vi "定点周期设置.vi"(7 "Display State In":T1={"仪器状态"=FALSE, "仪器时间"=timestamp(0 s since 1904-01-01), "测量参数"={"氨氮"=TRUE, "总磷"=TRUE, "总氮"=TRUE, "CODMn"=TRUE, "CODCr"=FALSE}, "调用模块名称"="", "测试状态"={"启动时间"=timestamp(0 s since 1904-01-01), "结束时间"=timestamp(0 s since 1904-01-01), "启动次数"=0.0}}, 9 "间隔启动":T7, 10 "定点周期":T4, 11 "周期模式":T3) -> (2 "保存输出":bool, 3 "周期设置输出":T6={"周期模式"=enum."不启用", "测量参数"={"氨氮"=TRUE, "总磷"=TRUE, "总氮"=TRUE, "CODMn"=TRUE, "CODCr"=FALSE}, "定点周期"={"启动命令"=enum."", "启动命令 2"=enum."", "启动命令 3"=enum."", "启动命令 4"=enum."", "启动命令 5"=enum."", "启动命令 6"=enum."", "启动命令 7"=enum."", "启动命令 8"=enum."", "启动命令 9"=enum."", "启动命令 10"=enum."", "启动命令 11"=enum."", "启动命令 12"=enum."", "启动命令 13"=enum."", "启动命令 14"=enum."", "启动命令 15"=enum."", "启动命令 16"=enum."", "启动命令 17"=enum."", "启动命令 18"=enum."", "启动命令 19"=enum."", "启动命令 20"=enum."", "启动命令 21"=enum."", "启动命令 22"=enum."", "启动命令 23"=enum."", "启动命令 24"=enum.""}, "间隔设置"={"启动命令"=enum."", "启动间隔"=0.0, "启动次数"=0}})   [LabVIEW 2016, in "ZK定时设置.xctl"]
panel:
  out "测试状态.结束时间":timestamp caption="结束时间" format="%<%y/%m/%d %H:%M:%S>T"
  out "测试状态.启动次数":dbl caption="启动次数"
  out "测试状态.启动时间":timestamp caption="启动时间" format="%<%y/%m/%d %H:%M:%S>T"
  in  "测量参数":T2={"氨氮"=TRUE, "总磷"=TRUE, "总氮"=TRUE, "CODMn"=TRUE, "CODCr"=FALSE}
  in  "保存":bool
  in  "退出":bool
  in  "批量设置":bool
  out "周期模式选择卡":enum32{"选项卡 1", "选项卡 2"}(tab)
  # "分钟"
  # "次"
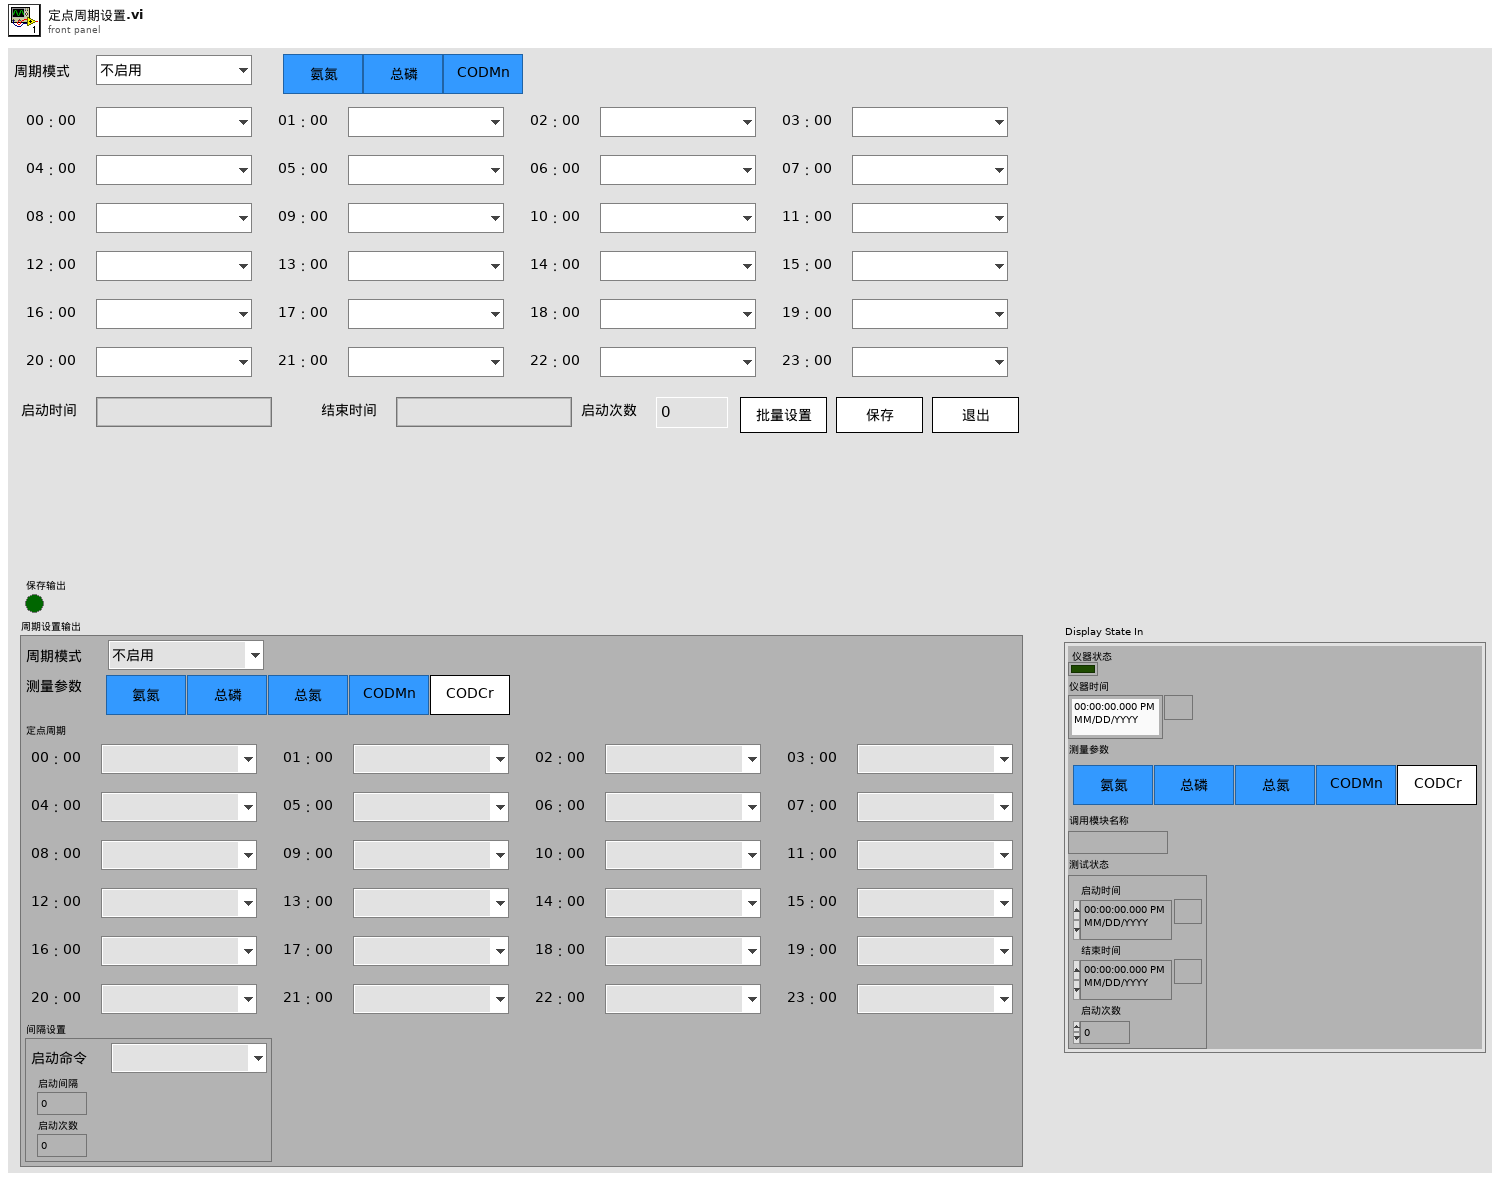
[diagram p1: front panel]
types:
  T1 = typedef "ZK定时设置.xctl/状态 1.ctl" = cluster{"仪器状态":bool, "仪器时间":timestamp, "测量参数":T2, "调用模块名称":string, "测试状态":cluster{"启动时间":timestamp, "结束时间":timestamp, "启动次数":dbl}}
  T2 = typedef "ZK定时设置.xctl/测量参数.ctl" = cluster{"氨氮":bool, "总磷":bool, "总氮":bool, "CODMn":bool, "CODCr":bool}
  T3 = typedef "ZK定时设置.xctl/周期模式设置.ctl" = enum16{"不启用", "定点模式", "间隔模式"}
  T4 = typedef "ZK定时设置.xctl/定点周期设置.ctl" = cluster{"启动命令":T5, "启动命令 2":T5, "启动命令 3":T5, "启动命令 4":T5, "启动命令 5":T5, "启动命令 6":T5, "启动命令 7":T5, "启动命令 8":T5, "启动命令 9":T5, "启动命令 10":T5, "启动命令 11":T5, "启动命令 12":T5, "启动命令 13":T5, "启动命令 14":T5, "启动命令 15":T5, "启动命令 16":T5, "启动命令 17":T5, "启动命令 18":T5, "启动命令 19":T5, "启动命令 20":T5, "启动命令 21":T5, "启动命令 22":T5, "启动命令 23":T5, "启动命令 24":T5}
  T5 = typedef "ZK定时设置.xctl/启动命令选择.ctl" = enum16{"", "加标回收（启动采配水）", "加标回收（不启动采配水）", "水样测试（启动采配水）", "水样测试（不启动采配水）", "平行样测试（启动采配水）", "平行样测试（不启动采配水）", "集成干预测试"}
  T6 = cluster{"周期模式":T3, "测量参数":T2, "定点周期":T4, "间隔设置":cluster{"启动命令":T5, "启动间隔":dbl, "启动次数":i32}}
  T7 = typedef "ZK定时设置.xctl/间隔启动设置.ctl" = cluster{"启动命令":T5, "启动间隔":dbl, "启动次数":i32}
  T8 = typedef "周期设置.lvlib/周期模式设置.ctl" = enum16{"不启用", "定点模式", "间隔模式"}
  T9 = cluster{"周期模式":T3, "测量参数":T2, "定点周期":T4, cluster{"启动命令":T5, "启动间隔":dbl, "启动次数":i32}}
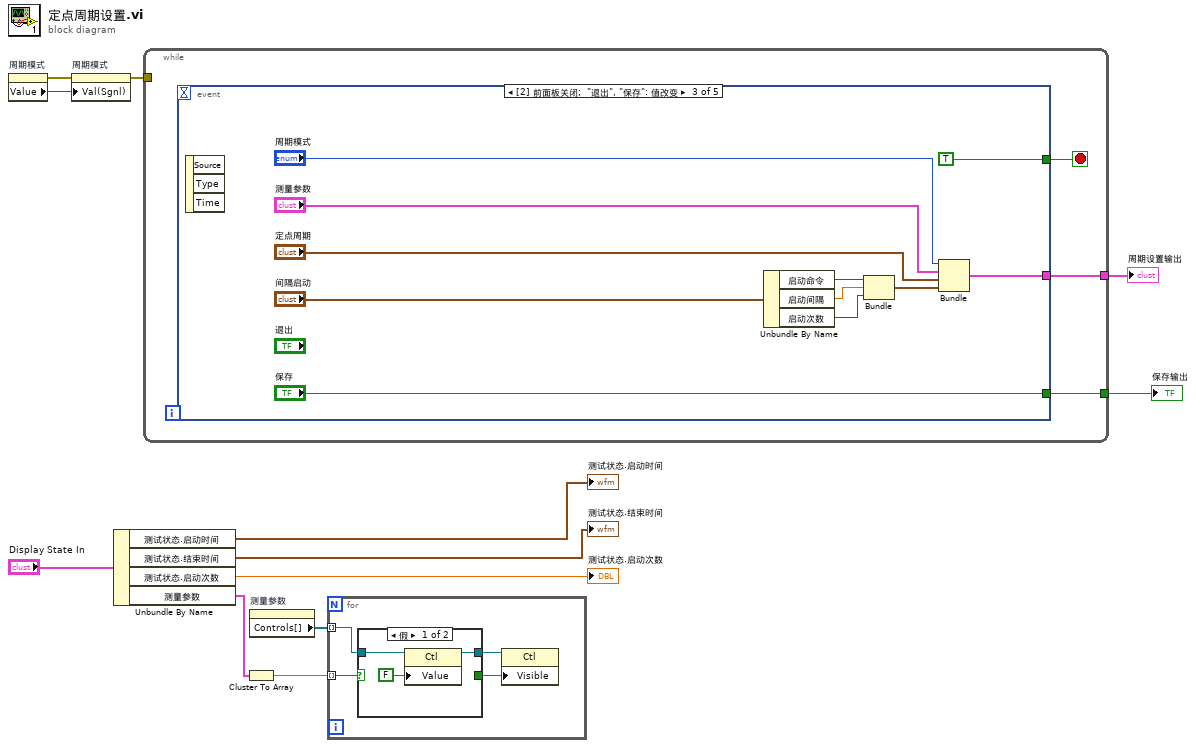
[diagram p0: block diagram]
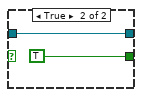
[diagram p2: hidden frame]
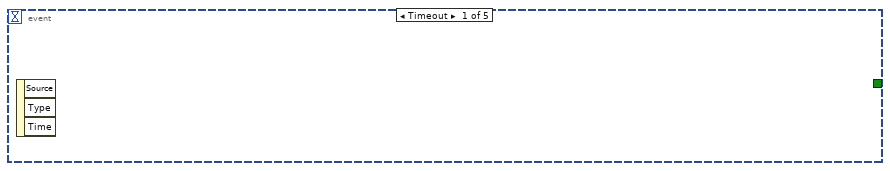
[diagram p3: hidden frame]
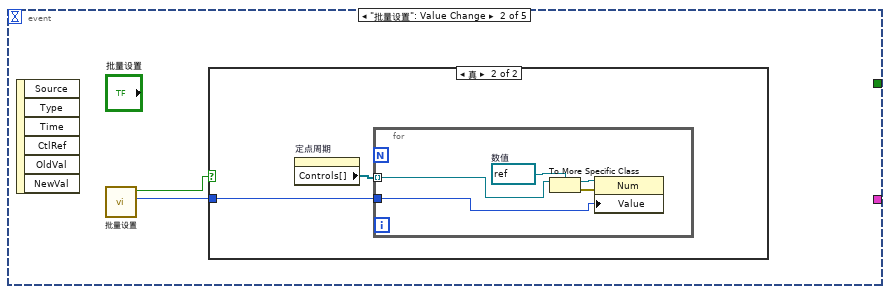
[diagram p4: hidden frame]
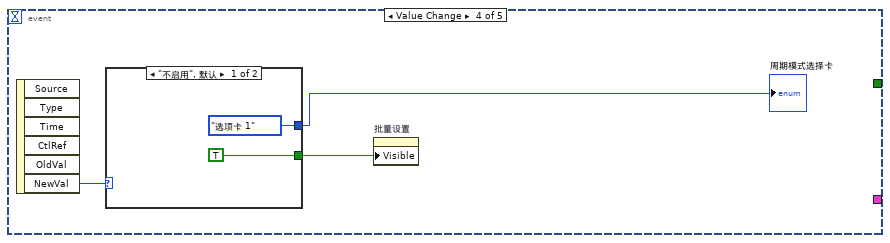
[diagram p6: hidden frame]
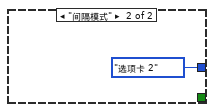
[diagram p7: hidden frame]
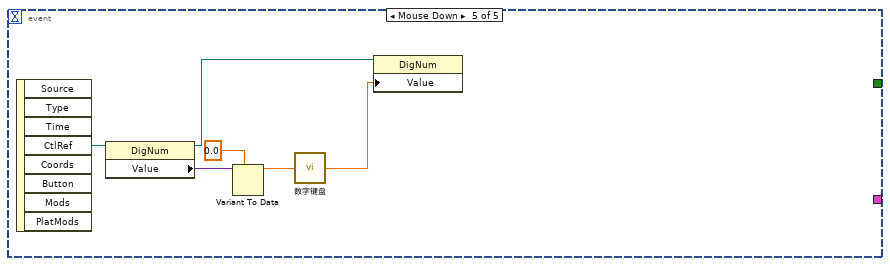
[diagram p8: hidden frame]
diagram:
  n1 = property on="周期模式" class="Enum (严格)"() -> (error out=w11:errorcluster, "Value"=w12:T8)  [unwired: 2 in, 1 out]
  n2 = property on="周期模式" class="Enum (严格)"(error in=w11, "Val(Sgnl)"=w12) -> (error out=w10:errorcluster)  [unwired: 1 in, 1 out]
  n3 = Unbundle By Name("Display State In") -> ("测试状态.启动时间"=→"测试状态.启动时间":timestamp, "测试状态.结束时间"=→"测试状态.结束时间":timestamp, "测试状态.启动次数"=→"测试状态.启动次数":dbl, "测量参数"=w1:T2)
  n4 = while {
    tunnel: [w14] -> w9
    tunnel: w10 -> [_]
    tunnel: [w13] -> w8
    stop <- w15 stop-if-true
    n5 = event shown="[2] 前面板关闭;  \"退出\", \"保存\": 值改变" {
      selector: _ -> [_ _ _ _ _]
      dyn-events: _ -> [_ _ _ _ _]
      timeout: _ -> [_ _ _ _ _]
      tunnel: [_ _ TRUE _ _] -> w15
      tunnel: [_ _ w34 _ _] -> w14
      tunnel: [_ _ "保存" _ _] -> w13
      event Timeout {
        n6 = event-data() -> ()  [unwired: 1 in, 3 out]
      }
      event "批量设置": Value Change {
        n7 = event-data() -> ()  [unwired: 1 in, 6 out]
        n8 = call "批量设置.vi"() -> ("启动命令 2"=w17:T5, "确定 2"=w16:bool)  [unwired: 10 in]
        n9 = case shown="真" w16 {
          tunnel: w17 -> [_ w18]
          frame False {
          }
          frame True {
            n10 = property on="定点周期" class="Clust (严格)"() -> ("Controls[]"=w19:refnum<vi>[])  [unwired: 2 in, 2 out]
            n11 = for {
              tunnel: w19 -> [w24] mode=indexing
              tunnel: w18 -> [w20]
              w23 = refnum<vi> refnum  # 数值
              n12 = To More Specific Class(target class=w23, reference=w24) -> (specific class reference=w22:refnum<vi>, error out=w21:errorcluster)  [unwired: 1 in]
              n13 = property class="Num"(reference=w22, error in=w21, "Value"=w20) -> ()  [unwired: 2 out]
            }
          }
        }
      }
      event Panel Close; "退出", "保存": Value Change {
        n14 = event-data() -> ()  [unwired: 1 in, 3 out]
        n15 = Unbundle By Name("间隔启动") -> ("启动命令"=w31:T5, "启动间隔"=w30:dbl, "启动次数"=w29:i32)
        n16 = Bundle("启动命令"=w31, "启动间隔"=w30, "启动次数"=w29) -> (w28:cluster{"启动命令":T5, "启动间隔":dbl, "启动次数":i32})  [unwired: 1 in]
        n17 = Bundle("周期模式"="周期模式", "测量参数"="测量参数", "定点周期"="定点周期", w28) -> (w34:T9)  [unwired: 1 in]
      }
      event Value Change {
        n18 = event-data() -> ("NewVal"=w37:T3)  [unwired: 1 in, 5 out]
        n19 = case shown="\"不启用\", 默认" w37 {
          tunnel: [TRUE ("可见") _] -> w38
          tunnel: [enum32{"选项卡 1", "选项卡 2"}."选项卡 1" ("周期模式选择卡") enum32{"选项卡 1", "选项卡 2"}."选项卡 2" ("周期模式选择卡")] -> w36
          frame "不启用", Default {
          }
          frame "间隔模式" {
          }
        }
        "周期模式选择卡" <- w36
        n20 = property on="批量设置" class="Bool"("Visible"=w38) -> ()  [unwired: 2 in, 2 out]
      }
      event Mouse Down {
        n21 = event-data() -> ("CtlRef"=w47:refnum<vi>)  [unwired: 1 in, 7 out]
        n22 = property class="DigNum"(reference=w47) -> (reference out=w46:refnum<vi>, "Value"=w45:variant)  [unwired: 1 in, 1 out]
        n23 = Variant To Data(type=0.0, Variant=w45) -> (data=w43:dbl)  [unwired: 1 in, 1 out]
        n24 = call "数字键盘.vi"("OldNumber"=w43) -> ("NewNumber"=w42:sgl)
        n25 = property class="DigNum"(reference=w46, "Value"=w42) -> ()  [unwired: 1 in, 2 out]
      }
    }
  }
  "周期设置输出" <- w9
  "保存输出" <- w8
  n26 = Cluster To Array(cluster=w1) -> (array=w2:bool[])
  n27 = property on="测量参数" class="Clust (严格)"() -> ("Controls[]"=w3:refnum<vi>[])  [unwired: 2 in, 2 out]
  n28 = for {
    tunnel: w3 -> [w49] mode=indexing
    tunnel: w2 -> [w51] mode=indexing
    n29 = case shown="假" w51 {
      tunnel: [w53 w56] -> w50
      tunnel: w49 -> [w54 w56]
      tunnel: [_ TRUE ("可见")] -> w48
      frame False {
        n30 = property class="Ctl"(reference=w54, "Value"=FALSE) -> (reference out=w53:refnum<vi>)  [unwired: 1 in, 1 out]
      }
      frame True {
      }
    }
    n31 = property class="Ctl"(reference=w50, "Visible"=w48) -> ()  [unwired: 1 in, 2 out]
  }
